vi "Wooden Clock.vi"() -> ()   [LabVIEW 2012]
panel:
  out "H":dbl(knob) scale=0.0..12.0
  out "M":dbl(knob) scale=0.0..60.0
  out "S":dbl(knob) scale=0.0..12.0
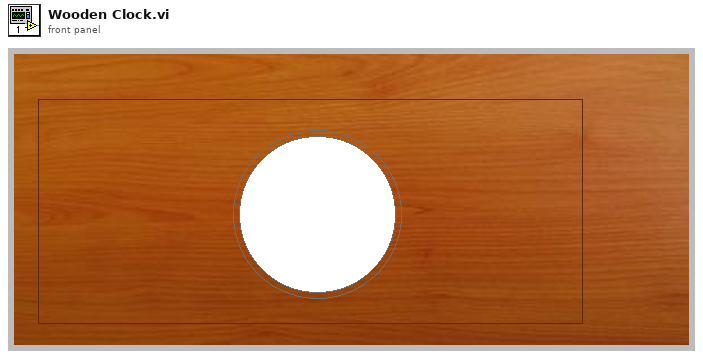
[diagram p1: front panel]
types:
  T1 = cluster{"second":i32, "minute":i32, "hour":i32, "day of month":i32, "month":i32, "year":i32, "day of week":i32, "day of year":i32, "is DST":i32}
  T2 = cluster{"second":dbl, "minute":dbl, "hour":dbl, "day of month":dbl, "month":dbl, "year":dbl, "day of week":dbl, "day of year":dbl, "is DST":dbl}
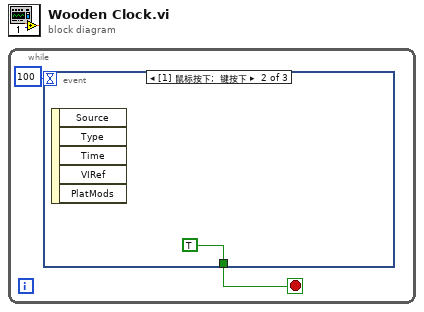
[diagram p0: block diagram]
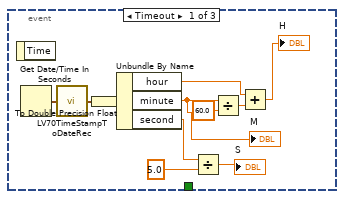
[diagram p2: hidden frame]
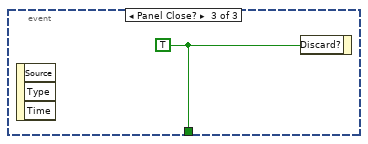
[diagram p3: hidden frame]
diagram:
  n1 = while {
    stop <- w1 stop-if-true
    n2 = event shown="[1] 鼠标按下;  键按下" {
      selector: _ -> [_ _ _]
      dyn-events: _ -> [_ _ _]
      timeout: 100 -> [_ _ _]
      tunnel: [_ TRUE w15] -> w1
      event Timeout {
        n3 = event-data() -> ()  [unwired: 1 in, 1 out]
        n4 = Get Date/Time In Seconds() -> (seconds since 1Jan1904=w13:timestamp)
        n5 = call <vilib>:"LV70TimeStampToDateRec.vi"("time stamp"=w13) -> ("date time rec"=w12:T1)
        n6 = To Double Precision Float(number=w12) -> (double precision float=w7:T2)
        n7 = Unbundle By Name(w7) -> ("hour"=w8:dbl, "minute"=w3:dbl, "second"=w4:dbl)
        "M" <- w3
        n8 = Divide(x=w4, y=5.0) -> (x/y=→"S":dbl)
        n9 = Divide(x=w3, y=60.0) -> (x/y=w9:dbl)
        n10 = Add(x=w8, y=w9) -> (x+y=→"H":dbl)
      }
      event Mouse Down; Key Down {
        n11 = event-data() -> ()  [unwired: 1 in, 5 out]
      }
      event Panel Close? {
        w15 = TRUE
        n12 = event-data() -> ()  [unwired: 1 in, 3 out]
        n13 = event-data("Discard?"=w15) -> ()  [unwired: 1 in, 1 out]
      }
    }
  }
